vi "Add_Subscriber.vi"(8 "error in (no error)":errorcluster, 11 "Add_subscriber":T1={"value"="11111111111111111111111111111111", "Add_Subscriber"="//add_subscriber", "N"=1, "imsi"="10.2.0.1", "phone_no"=0, "key_value"="8baf473f2f8fd09487cccbd7097c6862", "op/opc_value"="opc", "mnc-length"="00"} {"phone_no" min=0 max=2; "N" min=1 max=2}) -> (0 "error out":errorcluster, 3 "Output String":string)   [LabVIEW 2021]
uses:
  Controls/TCP_FGV.ctl
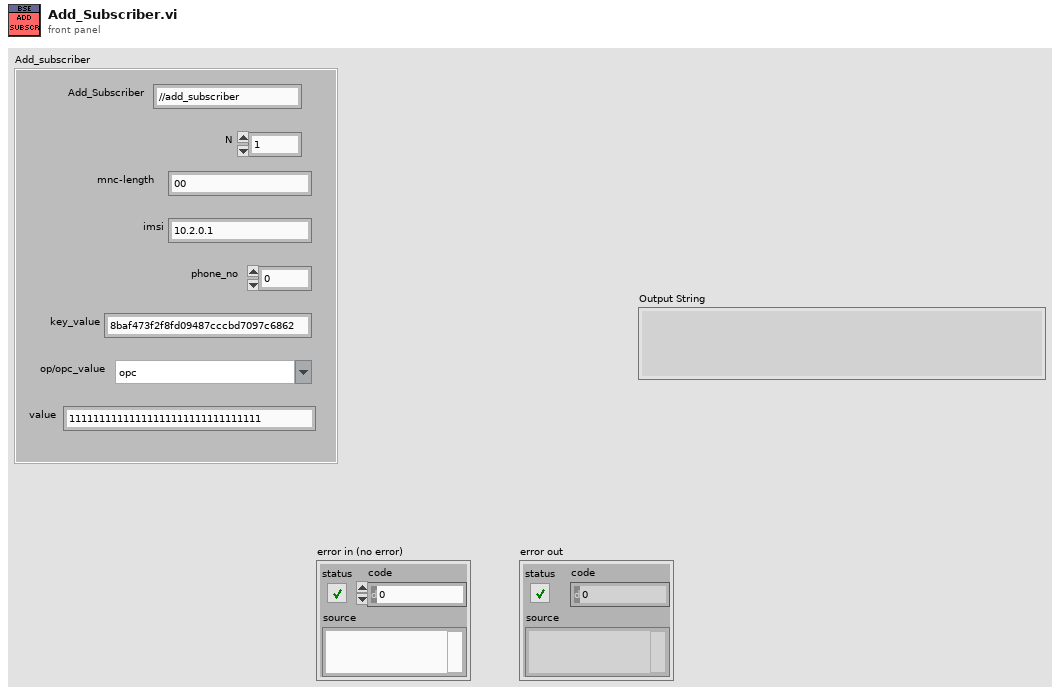
[diagram p1: front panel]
types:
  T1 = cluster{"value":string, "Add_Subscriber":string, "N":i32, "imsi":string, "phone_no":i32, "key_value":string, "op/opc_value":string, "mnc-length":string}
  T2 = typedef "TCP_FGV.ctl" = enum16{"Open", "Read", "Write", "Close"}
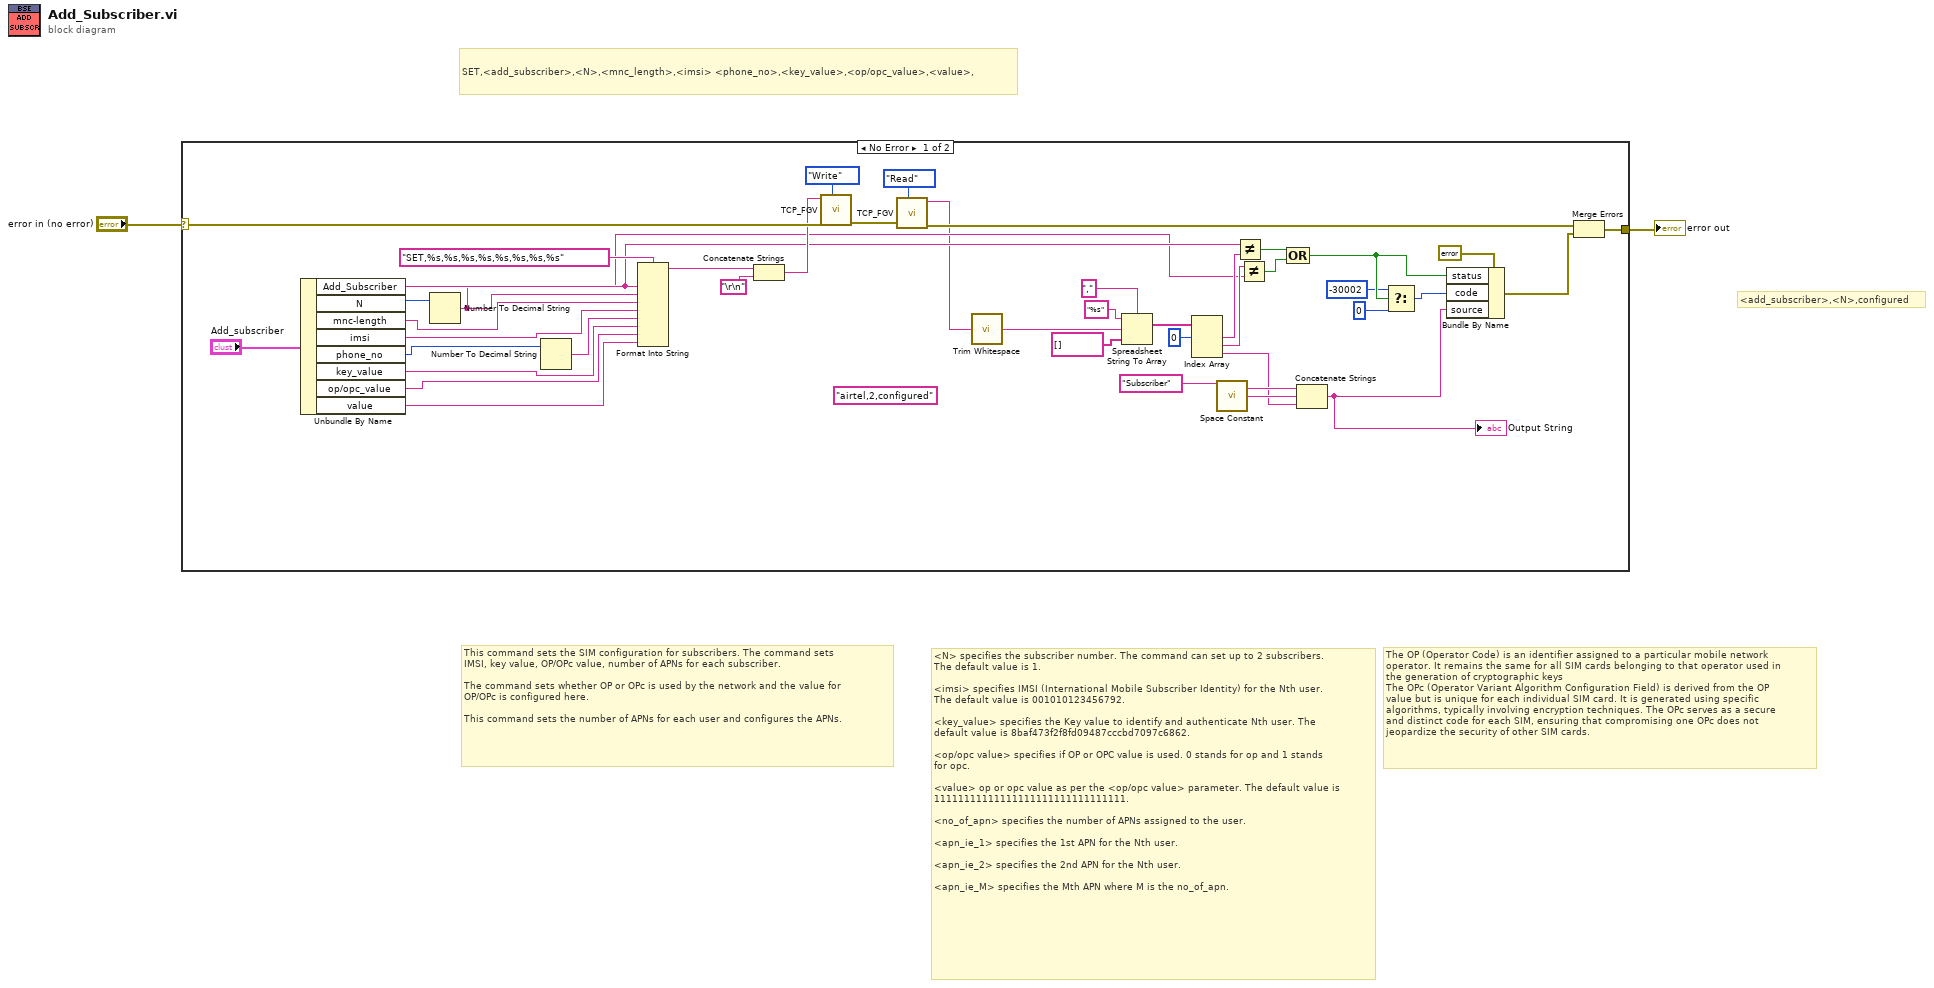
[diagram p0: block diagram]
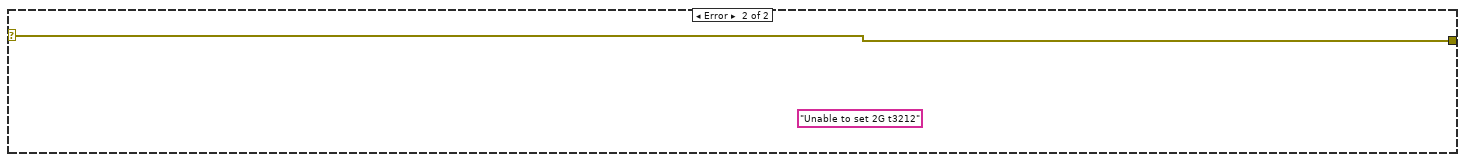
[diagram p2: hidden frame]
diagram:
  # "The OP (Operator Code) is an identifier assigned to a particular mobile network \noperator. It remains the same for all SIM cards belonging to that operator used in \nthe generation of cryptographic keys \nThe OPc (Operator Variant Algorithm Configuration Field) is derived from the OP \nvalue but is unique for each individual SIM card. It is generated using specific \nalgorithms, typically involving encryption techniques. The OPc serves as a secure\nand distinct code for each SIM, ensuring that compromising one OPc does not \njeopardize the security of other SIM cards."
  # "<N> specifies the subscriber number. The command can set up to 2 subscribers.  \nThe default value is 1. \n\n<imsi> specifies IMSI (International Mobile Subscriber Identity) for the Nth user. \nThe default value is 001010123456792. \n\n<key_value> specifies the Key value to identify and authenticate Nth user. The \ndefault value is 8baf473f2f8fd09487cccbd7097c6862.\n \n<op/opc value> specifies if OP or OPC value is used. 0 stands for op and 1 stands \nfor opc. \n \n<value> op or opc value as per the <op/opc value> parameter. The default value is \n11111111111111111111111111111111. \n\n<no_of_apn> specifies the number of APNs assigned to the user. \n\n<apn_ie_1> specifies the 1st APN for the Nth user. \n\n<apn_ie_2> specifies the 2nd APN for the Nth user. \n\n<apn_ie_M> specifies the Mth APN where M is the no_of_apn."
  # "SET,<add_subscriber>,<N>,<mnc_length>,<imsi> <phone_no>,<key_value>,<op/opc_value>,<value>,"
  # "This command sets the SIM configuration for subscribers. The command sets \nIMSI, key value, OP/OPc value, number of APNs for each subscriber. \n \nThe command sets whether OP or OPc is used by the network and the value for \nOP/OPc is configured here.  \n\nThis command sets the number of APNs for each user and configures the APNs."
  # "<add_subscriber>,<N>,configured"
  n1 = case shown="No Error" "error in (no error)" {
    selector: "error in (no error)" -> [w43 w45]
    tunnel: [w27 w45] -> w1
    frame No Error {
      (unwired) "airtel,2,configured" ("format string")
      n2 = Unbundle By Name("Add_subscriber") -> ("Add_Subscriber"=w16:string, "N"=w15:i32, "mnc-length"=w4:string, "imsi"=w5:string, "phone_no"=w14:i32, "key_value"=w13:string, "op/opc_value"=w12:string, "value"=w11:string)
      n3 = Number To Decimal String(number=w15) -> (decimal integer string=w9:string)  [unwired: 1 in]
      n4 = Number To Decimal String(number=w14) -> (decimal integer string=w18:string)  [unwired: 1 in]
      n5 = Format Into String(format string="SET,%s,%s,%s,%s,%s,%s,%s,%s", w16, w9, w4, w5, w18, w13, w12, w11) -> (resulting string=w23:string)  [unwired: 2 in, 1 out]
      n6 = Concatenate Strings(w23, "\r\n") -> (w22:string)
      n7 = call "TCP_FGV.vi"("Command"=w22, "error in (no error)"=w43, "Operation"=TCP_FGV."Write") -> ("error out"=w28:errorcluster)  [unwired: 6 in, 1 out]
      n8 = call "TCP_FGV.vi"("error in (no error)"=w28, "Operation"=TCP_FGV."Read") -> ("Data Out"=w3:string, "error out"=w30:errorcluster)  [unwired: 7 in]
      n9 = call <vilib>:"Trim Whitespace.vi"("string"=w3) -> ("trimmed string"=w40:string)  [unwired: 1 in]
      n10 = Spreadsheet String To Array(delimiter (Tab)=",", format string="%s", spreadsheet string=w40, array type (2D Dbl)=string[] []) -> (array=w37:string[])
      n11 = Index Array(array=w37, index #1=0 ("index")) -> (element #1=w19:string, element #2=w38:string, element #3=w6:string)  [unwired: 2 in]
      n12 = call <vilib>:"Space Constant.vi"() -> ("String"=w8:string)
      n13 = Not Equal?(x=w16, y=w19) -> (x != y?=w20:bool)
      n14 = Not Equal?(x=w38, y=w9) -> (x != y?=w39:bool)
      n15 = Compound Arithmetic op=OR(w20, w39) -> (w41:bool)
      n16 = Concatenate Strings("Subscriber" ("format string"), w8, w6) -> (w26:string)
      "Output String" <- w26
      n17 = Select(t=-30002 ("code"), s=w41, f=0 ("code")) -> (s? t:f=w42:i32)
      n18 = Bundle By Name(cluster=errorcluster {"status"=FALSE, "code"=0, "source"=""} ("error constant"), "status"=w41, "code"=w42, "source"=w26) -> (w29:errorcluster)
      n19 = Merge Errors(w30, w29) -> (w27:errorcluster)
    }
    frame Error {
      (unwired) "Unable to set 2G t3212" ("source")
    }
  }
  "error out" <- w1
